vi "RT Error Handler - System Health and FPGA Monitoring.vi"(4 "FPGA Error (FPGA)":errorcluster, 6 "Different Channel Count (FPGA)":bool, 8 "error in (no error)":errorcluster, 9 "DMA FIFO Full (FPGA)":bool, 10 "Module Underflow (FPGA)":bool, 11 "Message Queue":refnum<queue>) -> (3 "dup Message Queue":refnum<queue>)   [LabVIEW 2015]
uses:
  support/Message Queue/Message Cluster.ctl
  support/Message Queue/Message Queue.lvlib
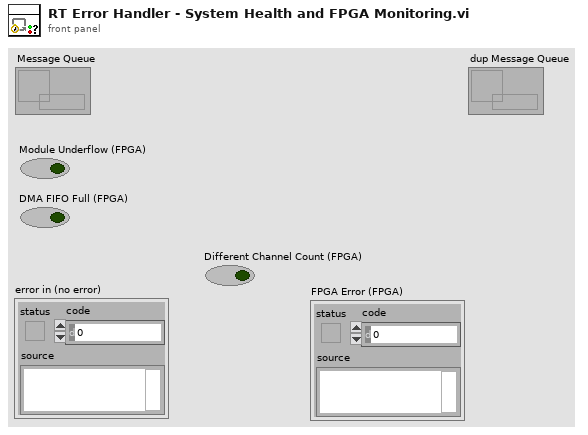
[diagram p1: front panel]
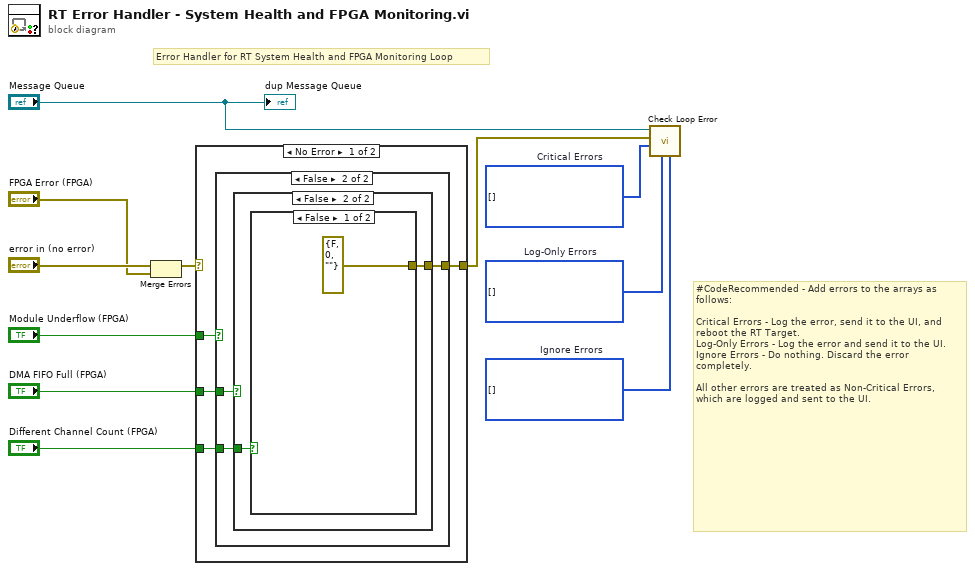
[diagram p0: block diagram]
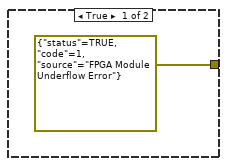
[diagram p2: hidden frame]
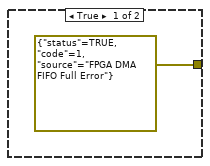
[diagram p3: hidden frame]
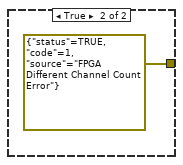
[diagram p4: hidden frame]
diagram:
  w9 = i32[] []  # Ignore Errors
  w10 = i32[] []  # Log-Only Errors
  w11 = i32[] []  # Critical Errors
  # "#CodeRecommended - Add errors to the arrays as follows:\n\nCritical Errors - Log the error, send it to the UI, and reboot the RT Target.\nLog-Only Errors - Log the error and send it to the UI.\nIgnore Errors - Do nothing. Discard the error completely.\n\nAll other errors are treated as Non-Critical Errors, which are logged and sent to the UI."
  # "Error Handler for RT System Health and FPGA Monitoring Loop"
  n1 = Merge Errors("error in (no error)", "FPGA Error (FPGA)") -> (w3:errorcluster)
  n2 = case shown="No Error" w3 {
    selector: w3 -> [_ w25]
    tunnel: "Module Underflow (FPGA)" -> [w15 _]
    tunnel: "DMA FIFO Full (FPGA)" -> [w13 _]
    tunnel: [w14 w25] -> w4
    tunnel: "Different Channel Count (FPGA)" -> [w12 _]
    frame No Error {
      n3 = case shown="False" w15 {
        tunnel: [errorcluster {"status"=TRUE, "code"=1, "source"="FPGA Module Underflow Error"} ("error constant") w19] -> w14
        tunnel: w13 -> [_ w18]
        tunnel: w12 -> [_ w17]
        frame True {
        }
        frame False {
          n4 = case shown="False" w18 {
            tunnel: [errorcluster {"status"=TRUE, "code"=1, "source"="FPGA DMA FIFO Full Error"} ("error constant") w22] -> w19
            tunnel: w17 -> [_ w21]
            frame True {
            }
            frame False {
              n5 = case shown="False" w21 {
                tunnel: [errorcluster {"status"=FALSE, "code"=0, "source"=""} ("error constant") errorcluster {"status"=TRUE, "code"=1, "source"="FPGA Different Channel Count Error"} ("error constant")] -> w22
                frame False {
                }
                frame True {
                }
              }
            }
          }
        }
      }
    }
    frame Error {
    }
  }
  n6 = call "Check Loop Error.vi"("Ignore Errors"=w9, "Log-Only Errors"=w10, "Critical Errors"=w11, "error to process"=w4, "Message Queue"="Message Queue") -> ()  [unwired: 5 in, 2 out]
  "dup Message Queue" <- "Message Queue"
